vi "EXAMPLE_PARSEFILE.vi"() -> ()   [LabVIEW 2014]
panel:
  in  "Listbox":i32(listbox)
  out "Variant":variant
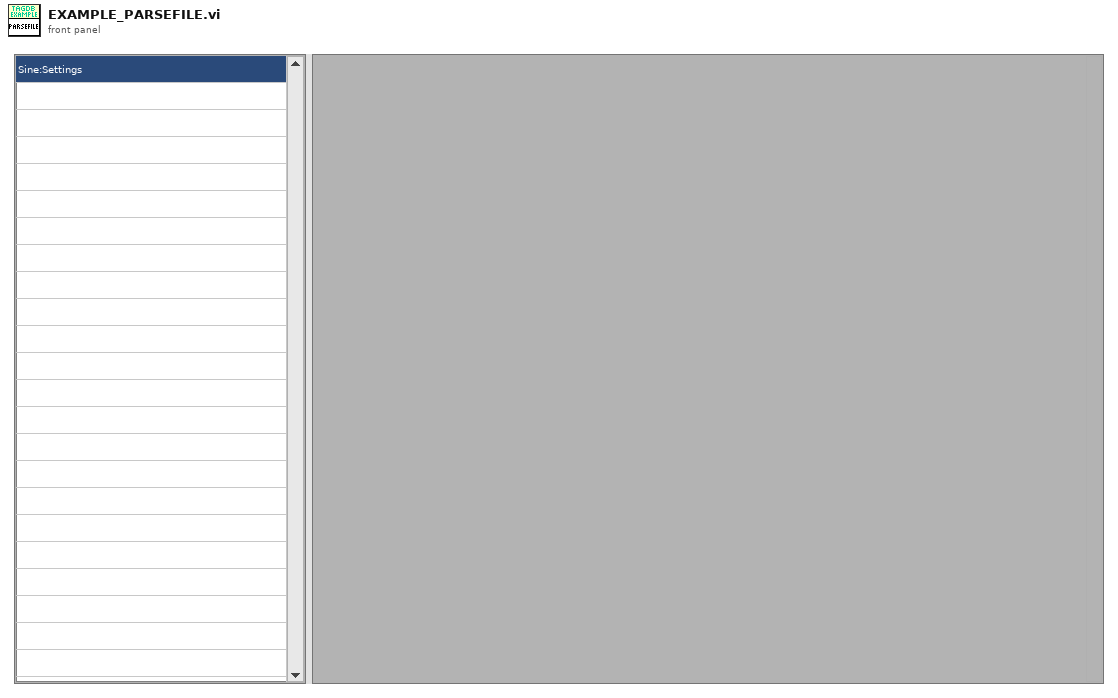
[diagram p1: front panel]
types:
  T1 = enum16{"open", "replace", "create", "open or create", "replace or create", "replace or create with confirmation"}
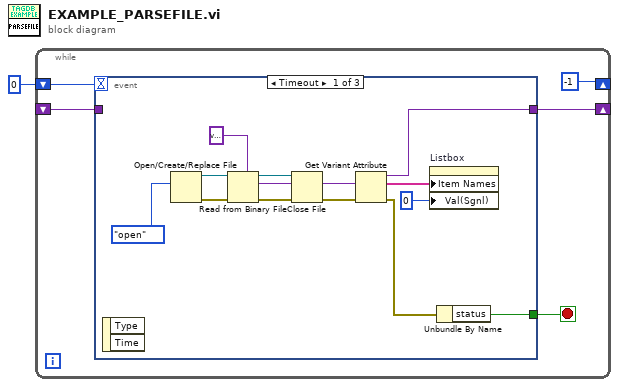
[diagram p0: block diagram]
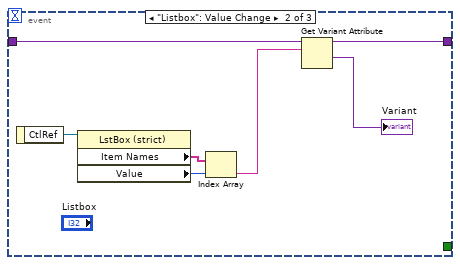
[diagram p2: hidden frame]
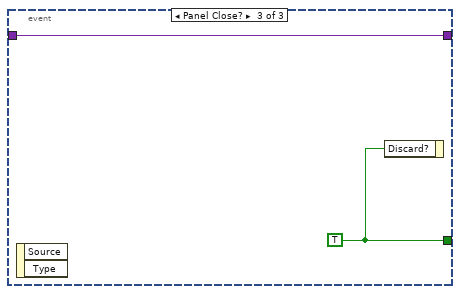
[diagram p3: hidden frame]
diagram:
  n1 = while {
    shift-right: [-1] -> _
    shift-left: 0 -> [w5]
    shift-right: [w3] -> _
    shift-left: _ -> [w2]
    stop <- w6 stop-if-true
    n2 = event shown="[0] Timeout" {
      selector: _ -> [_ _ _]
      dyn-events: _ -> [_ _ _]
      timeout: w5 -> [_ _ _]
      tunnel: [w7 _ w28] -> w6
      tunnel: [w11 w21 w27] -> w3
      tunnel: w2 -> [_ w23 w27]
      event Timeout {
        n3 = event-data() -> ()  [unwired: 1 in, 2 out]
        n4 = Open/Create/Replace File(operation (0:open)=T1."open") -> (refnum out=w14:refnum<file>, error out=w15:errorcluster)  [unwired: 5 in, 1 out]
        n5 = Read from Binary File(5:variant ("Variant"), 8:w15, 11:w14) -> (0:w13:errorcluster, 2:w18:variant, 3:w12:refnum<file>)  [unwired: 3 in, 1 out]
        n6 = Close File(refnum=w12, error in=w13) -> (error out=w19:errorcluster)  [unwired: 1 out]
        n7 = Get Variant Attribute(Variant=w18, error in=w19) -> (duplicate Variant=w11:variant, names=w10:string[], error out=w8:errorcluster)  [unwired: 2 in, 1 out]
        n8 = property on="Listbox" class="LstBox (strict)"("Item Names"=w10, "Val(Sgnl)"=0 ("Value (Signaling)")) -> ()  [unwired: 2 in, 2 out]
        n9 = Unbundle By Name(w8) -> ("status"=w7:bool)
      }
      event "Listbox": Value Change {
        n10 = event-data() -> ("CtlRef"=w26:refnum<vi>)  [unwired: 1 in]
        n11 = property class="LstBox (strict)"(reference=w26) -> ("Item Names"=w24:string[], "Value"=w25:i32)  [unwired: 1 in, 2 out]
        n12 = Index Array(array=w24, index=w25) -> (element=w22:string)
        n13 = Get Variant Attribute(Variant=w23, name=w22) -> (duplicate Variant=w21:variant, value=→"Variant":variant)  [unwired: 2 in, 2 out]
      }
      event Panel Close? {
        w28 = TRUE
        n14 = event-data() -> ()  [unwired: 1 in, 2 out]
        n15 = event-data("Discard?"=w28) -> ()  [unwired: 1 in, 1 out]
      }
    }
  }
